vi "Write To Symbol.vi"() -> ()   [LabVIEW 2018]
uses:
  TwinCAT ADS Class/TwinCAT ADS.lvclass
panel:
  in  "HTTP Request Messages":T1(array[cluster])=[{"Request Line"={"Method"=0, "URI"="/images/cats.html", "Protocol"="HTTP/1.1"}, "Header Fields"={"Host"="www.animals.com", "Accept"="image/gif image/jpeg", "Accept-Language"="en-GB", "Accept-Encoding"="gzip, deflate", "User-Agent"="Mozilla/5.0"}}, {"Request Line"={"Method"=0, "URI"="/pages/dogs.html", "Protocol"="HTTP/1.1"}, "Header Fields"={"Host"="www.animals.com", "Accept"="*/*", "Accept-Language"="en-US,en;q=0.9", "Accept-Encoding"="gzip, deflate", "User-Agent"="Chrome/100.0.4896.60"}}, {"Request Line"={"Method"=0, "URI"="/Identity/Dropdown?n=...", "Protocol"="HTTP/1.1"}, "Header Fields"={"Host"="www.bing.com", "Accept"="text/html text/plain image/gif image/jpeg", "Accept-Language"="en-US,en;q=0.9", "Accept-Encoding"="gzip, deflate, br", "User-Agent"="Edge/100.0.1185.29"}}] {"Request Line"."Method" items=["GET", "HEAD", "POST", "PUT", "DELETE", "CONNECT", "OPTIONS"]}
  # "Example PLC Source Code is available at:\nhttps://github.com/fisothemes/LabVIEW-TwinCAT-ADS/tree/master/src/PLC"
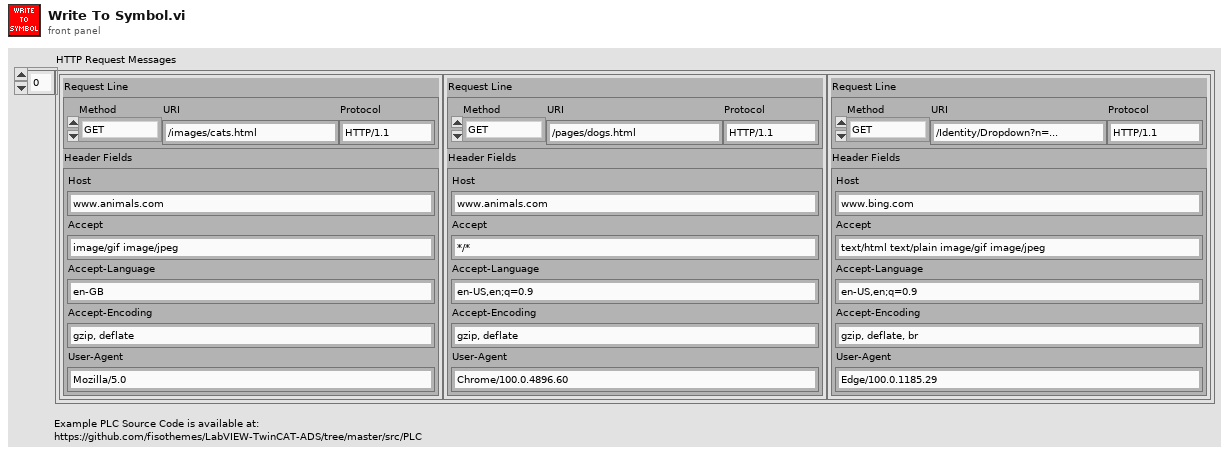
[diagram p1: front panel]
types:
  T1 = cluster{"Request Line":cluster{"Method":u16, "URI":string, "Protocol":string}, "Header Fields":cluster{"Host":string, "Accept":string, "Accept-Language":string, "Accept-Encoding":string, "User-Agent":string}}[]
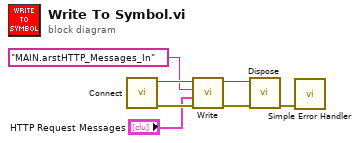
[diagram p0: block diagram]
diagram:
  n1 = call "Connect.vi"() -> ("error out"=w7:errorcluster, "TwinCAT ADS out"=w6:refnum<class "TwinCAT ADS.lvclass">)  [unwired: 10 in]
  n2 = call "Write.vi"("error in (no error)"=w7, "Value"="HTTP Request Messages", "Symbol Name"="MAIN.arstHTTP_Messages_In" ("Name"), "TwinCAT ADS in"=w6) -> ("error out"=w5:errorcluster, "TwinCAT ADS out"=w4:refnum<class "TwinCAT ADS.lvclass">)  [unwired: 6 in]
  n3 = call "Dispose.vi"("error in (no error)"=w5, "TwinCAT ADS in"=w4) -> ("error out"=w1:errorcluster)  [unwired: 9 in]
  n4 = call <vilib>:"Simple Error Handler.vi"("error in (no error)"=w1) -> ()  [unwired: 4 in, 5 out]
